vi "PH_Timing.PC link SRDG Channel Infos.vi"(0 "i ref in":refnum<vi>, 1 "data":i8[](array[numeric]), 2 "Service Name":string="N/A", 3 "typeDescriptor":string="D:N", 4 "no link":bool, 5 "error in":errorcluster) -> (14 "i ref out":refnum<vi>, 19 "error out":errorcluster)   [LabVIEW 2014, in "PH_Timing.lvlib"]
doc: "This VI writes the incoming information to own attributes and sets GUI elements."
uses:
  PH_Timing.lvlib
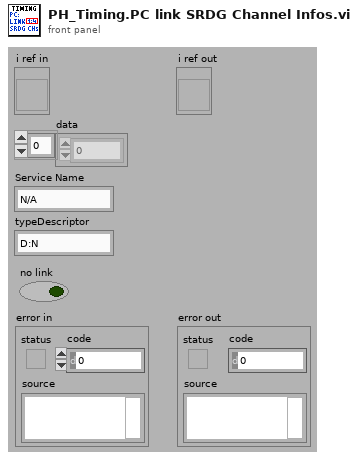
[diagram p1: front panel]
types:
  T1 = typedef "PH_Timing.lvlib/PH_Timing.i attribute.ctl" = cluster{"Sequencer":cluster{"linked?":bool, "Proc State":string, "Ref State":refnum<vi>}, "Gate Generator":cluster{"GD":cluster{"Device Status":T2, "linked?":bool}, "Settings":T3, "GUI Ref":refnum<vi>}, "Interlock Bypass":cluster{"Instancename":string, "Switch linked?":bool, "Device Status":T2, "Ref Status":refnum<vi>}, "Roughtuner":cluster{"Settings":T4, "GUI Ref":refnum<vi>, "GD":cluster{"Device Status":T2, "linked?":bool}}, "0,5Hz Gater":cluster{"Settings":T5, "GUI Ref":refnum<vi>, "GD":cluster{"Device Status":T2, "linked?":bool}}, "Slow Trigger":cluster{"Settings":T6, "GUI Ref":refnum<vi>, "Service ID Delay":i32, "Service ID Ext Trig":i32, "Wanted Settings":T6}, "Timing Mode":cluster{"Mode":T7, "GUI Ref":refnum<vi>, "Service ID T2":i32, "Service ID Mode":i32, "Wanted Mode":T7}, "ns Generator":cluster{"Settings":T8, "ns Generator Settings":refnum<vi>, "GD":cluster{"Device Status":T2, "linked?":bool}}, "Phase FEs":cluster{"Settings":T11, "GUI Ref":refnum<vi>, "Service ID Phase":i32, "Wanted Settings":T11}, "GD GUI Refs":refnum<vi>[], "Heads":T12[], "GUI Ref Delete":refnum<vi>}
  T2 = typedef "PH_StatusHandler.lvlib/PH_StatusHandler.Status.ctl" = i16
  T3 = typedef "PH_Timing.lvlib/PH_Timing.GateGen.ctl" = cluster{"Instance":string, "Channel Gate":i32, "Channel T2":i32, "Width Gate":dbl, "Width T2":dbl, "Delay Gate":dbl, "Delay T2":dbl, "Gate activ":bool, "T2 activ":bool, "System Mode":enum16{"Normal", "Single", "Burst", "Duty Cycle"}}
  T4 = typedef "PH_Timing.lvlib/PH_Timing.Roughtuner.ctl" = cluster{"Instance":string, "Phase PHELIX / UNILAC":cluster{"Channel":u16, "relative to":u16, "Delay [ms]":dbl}, "Pulse Length":cluster{"Channel":u16, "relative to":u16, "Delay [ms]":dbl}, "Trigger":cluster{"externally?":bool, "Rate [Hz]":dbl}}
  T5 = typedef "PH_Timing.lvlib/PH_Timing.0.5HzGater.ctl" = cluster{"Instance":string, "Channel ns FE Delay":i32, "Channel 0.5Hz":i32, "Width ns FE Delay":dbl, "Width 0.5Hz":dbl, "Delay ns FE Delay":dbl, "Delay 0.5Hz":dbl, "ns FE Delay active":bool, "0.5Hz activ":bool, "ns FE Delay inverted":bool, "0.5Hz inverted":bool}
  T6 = typedef "PH_Timing.lvlib/PH_Timing.Slow Trigger Settings.ctl" = cluster{"Delay":dbl, "externally triggered?":bool}
  T7 = typedef "PH_Timing.lvlib/PH_Timing.Timing Mode.ctl" = cluster{"T2":i16, "Modeselector":enum32{"10 Hz", "0.5 Hz", "Shot"}}
  T8 = typedef "PH_Timing.lvlib/PH_Timing.ns Generator.ctl" = cluster{"Instance":string, "Phase fs / ns FE":cluster{"Channel":T9, "Settings":T10}}
  T9 = typedef "Stanford Research DG645 - Driver.lvlib/Channel.ctl" = i32
  T10 = typedef "PH_SRDG645.lvlib/PH_SRDG645.Channel Settings.ctl" = cluster{"Delay [s]":dbl, "relative to":i32}
  T11 = typedef "PH_Timing.lvlib/PH_Timing.Phase FEs.ctl" = cluster{"Phase":dbl}
  T12 = typedef "PH_Timing.lvlib/PH_Timing.PU Data.ctl" = cluster{"linked?":bool, "Data":T13, "GD":cluster{"Device Status":T2, "linked?":bool}, "GUI Ref":refnum<vi>, "PU":T14}
  T13 = typedef "PH_Timing.lvlib/PH_Timing.PU Info.ctl" = cluster{"Act CH?":bool, "GD":string, "CH":i32, "Delay":dbl, "active":bool, "in Use?":bool}
  T14 = typedef "PH_PP_Common.lvlib/PH_PP_Common.PUs.ctl" = enum16{"no Info", "PA-19mm-1", "PA-19mm-2", "PA-45mm-PILC", "PA-45mm-MAIN", "MA-PU-1", "MA-PU-2", "MA-PU-3", "MA-PU-4", "MA-PU-5", "MA-PU-6", "MA-FR", "MA-PILC", "PA-45mm-DP"}
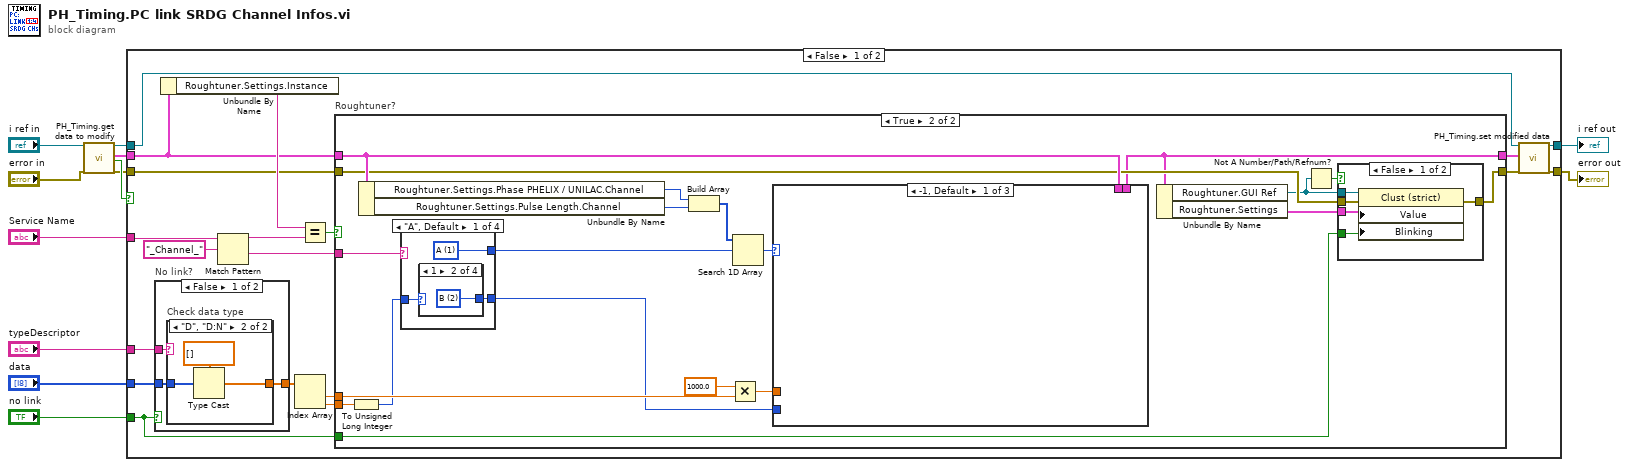
[diagram p0: block diagram]
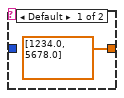
[diagram p2: hidden frame]
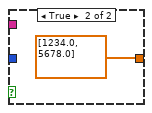
[diagram p3: hidden frame]
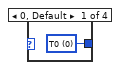
[diagram p6: hidden frame]
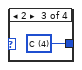
[diagram p7: hidden frame]
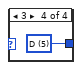
[diagram p8: hidden frame]
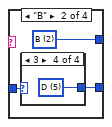
[diagram p9: hidden frame]
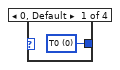
[diagram p10: hidden frame]
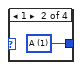
[diagram p11: hidden frame]
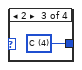
[diagram p12: hidden frame]
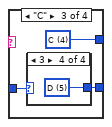
[diagram p13: hidden frame]
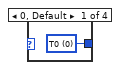
[diagram p14: hidden frame]
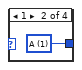
[diagram p15: hidden frame]
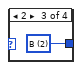
[diagram p16: hidden frame]
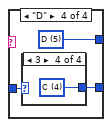
[diagram p17: hidden frame]
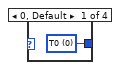
[diagram p18: hidden frame]
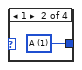
[diagram p19: hidden frame]
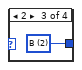
[diagram p20: hidden frame]
diagram:
  n1 = call "PH_Timing.get data to modify.vi"("i ref in"="i ref in", "error in (no error)"="error in") -> ("i ref out"=w4:refnum<vi>, "i attribute"=w9:T1, "timed out"=w10:bool, "error out"=w7:errorcluster)  [unwired: 14 in]
  n2 = case shown="False" w10 {
    tunnel: w4 -> [w13 w106]
    tunnel: [w31 w106] -> w5
    tunnel: w7 -> [w16 w105]
    tunnel: [w30 w105] -> w8
    tunnel: w9 -> [w14 _]
    tunnel: "no link" -> [w20 _]
    tunnel: "Service Name" -> [w29 _]
    tunnel: "data" -> [w26 _]
    tunnel: "typeDescriptor" -> [w25 _]
    frame False {
      n3 = case "No link?" shown="False" w20 {
        tunnel: [w34 dbl[] [1234.0, 5678.0]] -> w24
        tunnel: w26 -> [w33 _]
        tunnel: w25 -> [w32 _]
        frame False {
          n4 = case "Check data type" shown="\"D\", \"D:N\"" w32 {
            tunnel: [dbl[] [1234.0, 5678.0] w37] -> w34
            tunnel: w33 -> [_ w38]
            frame Default {
            }
            frame "D", "D:N" {
              n5 = Type Cast(type=dbl[] [], x=w38) -> (*(type *) &x=w37:dbl[])
            }
          }
        }
        frame True {
        }
      }
      n6 = Unbundle By Name(w14) -> ("Roughtuner.Settings.Instance"=w19:string)
      n7 = Match Pattern(string=w29, regular expression="_Channel_") -> (before substring=w18:string, after substring=w15:string)  [unwired: 1 in, 2 out]
      n8 = Index Array(array=w24) -> (element #1=w23:dbl, element #2=w22:dbl)  [unwired: 2 in]
      n9 = Equal?(x=w19, y=w18) -> (x = y?=w17:bool)
      n10 = case "Roughtuner?" shown="True" w17 {
        tunnel: w14 -> [w41 w49]
        tunnel: [w41 w45] -> w27
        tunnel: w23 -> [_ w58]
        tunnel: w22 -> [_ w52]
        tunnel: w16 -> [w40 w48]
        tunnel: [w40 w47] -> w21
        tunnel: w20 -> [_ w46]
        tunnel: w15 -> [_ w54]
        frame False {
        }
        frame True {
          n11 = To Unsigned Long Integer(number=w52) -> (unsigned 32bit integer=w51:u32)
          n12 = Unbundle By Name(w49) -> ("Roughtuner.Settings.Phase PHELIX / UNILAC.Channel"=w61:u16, "Roughtuner.Settings.Pulse Length.Channel"=w60:u16)
          n13 = case shown="\"A\", Default" w54 {
            tunnel: [w70 w77 w84 w91] -> w53
            tunnel: w51 -> [w69 w76 w83 w90]
            tunnel: [w68 w75 w82 w89] -> w50
            frame "A", Default {
              w70 = u16 1 items=["T0", "A", "B", "AB", "C", "D", "CD"] ("Channel")
              n14 = case shown="1" w69 {
                tunnel: [w71 w72 w73 w74] -> w68
                frame 0, Default {
                  w71 = u16 0 items=["T0", "A", "B", "AB", "C", "D", "CD"] ("Channel")
                }
                frame 1 {
                  w72 = u16 2 items=["T0", "A", "B", "AB", "C", "D", "CD"] ("Channel")
                }
                frame 2 {
                  w73 = u16 4 items=["T0", "A", "B", "AB", "C", "D", "CD"] ("Channel")
                }
                frame 3 {
                  w74 = u16 5 items=["T0", "A", "B", "AB", "C", "D", "CD"] ("Channel")
                }
              }
            }
            frame "B" {
              w77 = u16 2 items=["T0", "A", "B", "AB", "C", "D", "CD"] ("Channel")
              n15 = case shown="3" w76 {
                tunnel: [w78 w79 w80 w81] -> w75
                frame 0, Default {
                  w78 = u16 0 items=["T0", "A", "B", "AB", "C", "D", "CD"] ("Channel")
                }
                frame 1 {
                  w79 = u16 1 items=["T0", "A", "B", "AB", "C", "D", "CD"] ("Channel")
                }
                frame 2 {
                  w80 = u16 4 items=["T0", "A", "B", "AB", "C", "D", "CD"] ("Channel")
                }
                frame 3 {
                  w81 = u16 5 items=["T0", "A", "B", "AB", "C", "D", "CD"] ("Channel")
                }
              }
            }
            frame "C" {
              w84 = u16 4 items=["T0", "A", "B", "AB", "C", "D", "CD"] ("Channel")
              n16 = case shown="3" w83 {
                tunnel: [w85 w86 w87 w88] -> w82
                frame 0, Default {
                  w85 = u16 0 items=["T0", "A", "B", "AB", "C", "D", "CD"] ("Channel")
                }
                frame 1 {
                  w86 = u16 1 items=["T0", "A", "B", "AB", "C", "D", "CD"] ("Channel")
                }
                frame 2 {
                  w87 = u16 2 items=["T0", "A", "B", "AB", "C", "D", "CD"] ("Channel")
                }
                frame 3 {
                  w88 = u16 5 items=["T0", "A", "B", "AB", "C", "D", "CD"] ("Channel")
                }
              }
            }
            frame "D" {
              w91 = u16 5 items=["T0", "A", "B", "AB", "C", "D", "CD"] ("Channel")
              n17 = case shown="3" w90 {
                tunnel: [w92 w93 w94 w95] -> w89
                frame 0, Default {
                  w92 = u16 0 items=["T0", "A", "B", "AB", "C", "D", "CD"] ("Channel")
                }
                frame 1 {
                  w93 = u16 1 items=["T0", "A", "B", "AB", "C", "D", "CD"] ("Channel")
                }
                frame 2 {
                  w94 = u16 2 items=["T0", "A", "B", "AB", "C", "D", "CD"] ("Channel")
                }
                frame 3 {
                  w95 = u16 4 items=["T0", "A", "B", "AB", "C", "D", "CD"] ("Channel")
                }
              }
            }
          }
          n18 = Build Array(w61, w60) -> (w55:u16[])
          n19 = Multiply(x=1000.0, y=w58) -> (x*y=w56:dbl)
          n20 = Search 1D Array(1D array=w55, element=w53) -> (index of element=w59:i32)  [unwired: 1 in]
          n21 = case shown="-1, Default" w59 {
            tunnel: w56 -> [_ w97 w102]
            tunnel: w50 -> [_ w100 w104]
            tunnel: w49 -> [w96 w99 w103]
            tunnel: [w96 w98 w101] -> w45
            frame -1, Default {
            }
            frame 0 {
              n22 = Bundle By Name(cluster=w99, "Roughtuner.Settings.Phase PHELIX / UNILAC.Delay [ms]"=w97, "Roughtuner.Settings.Phase PHELIX / UNILAC.relative to"=w100) -> (w98:T1)
            }
            frame 1 {
              n23 = Bundle By Name(cluster=w103, "Roughtuner.Settings.Pulse Length.Delay [ms]"=w102, "Roughtuner.Settings.Pulse Length.relative to"=w104) -> (w101:T1)
            }
          }
          n24 = Unbundle By Name(w45) -> ("Roughtuner.GUI Ref"=w43:refnum<vi>, "Roughtuner.Settings"=w42:T4)
          n25 = Not A Number/Path/Refnum?(number/path/refnum=w43) -> (NaN/Path/Refnum?=w44:bool)
          n26 = case shown="False" w44 {
            tunnel: [w66 w67] -> w47
            tunnel: w48 -> [w65 w67]
            tunnel: w46 -> [w64 _]
            tunnel: w43 -> [w63 _]
            tunnel: w42 -> [w62 _]
            frame False {
              n27 = property class="Clust (strict)"(reference=w63, error in=w65, "Value"=w62, "Blinking"=w64) -> (error out=w66:errorcluster)  [unwired: 1 out]
            }
            frame True {
            }
          }
        }
      }
      n28 = call "PH_Timing.set modified data.vi"("i ref in"=w13, "i attribute"=w27, "error in (no error)"=w21) -> ("i ref out"=w31:refnum<vi>, "error out"=w30:errorcluster)  [unwired: 15 in]
    }
    frame True {
    }
  }
  "error out" <- w8
  "i ref out" <- w5
